vi "Read All FlexiFlow Device States--SubVI.vi"(8 "error in (no error)":errorcluster, 11 "Data Cluster in":T1 {"Flexi-Flow Devices"."Control State"."Control Mode" items=["Bus/RS232"=0, "FLOW-BUS slave"=2, "Valve close"=3, "Controller idle"=4, "Setpoint 100%"=7, "Valve fully open"=8, "Calibration mode"=9, "Setpoint 0%"=12, "RS232"=18, "Valve steering"=20, "Valve safe state"=22]}) -> (0 "error out":errorcluster, 3 "Data Cluster out":T1 {"Flexi-Flow Devices"."Control State"."Control Mode" items=["Bus/RS232"=0, "FLOW-BUS slave"=2, "Valve close"=3, "Controller idle"=4, "Setpoint 100%"=7, "Valve fully open"=8, "Calibration mode"=9, "Setpoint 0%"=12, "RS232"=18, "Valve steering"=20, "Valve safe state"=22]})   [LabVIEW 2025]
uses:
  phlair-shared-libraries/Modbus Flexi-Flow API/Bronkhorst Flexi-Flow ModbusTCP API.lvlib
  phlair-shared-libraries/Modbus Flexi-Flow API/Control Function Values--enum.ctl
  FlexiFlowInterface/Modbus Flexi-Flow Controls--cluster.ctl
  <vilib>/Plasmionique/MB Master/MB_Master_TCP/MB_Master_TCP.lvclass
  FlexiFlowInterface/Modbus Flexi-Flow Measure State--cluster.ctl
  FlexiFlowInterface/Modbus Flexi-Flow State--cluster.ctl
  FlexiFlowInterface/Module Data--cluster.ctl
  phlair-shared-libraries/Modbus Flexi-Flow API/Control Mode--enum.ctl
  FlexiFlowInterface/Device Type--enum.ctl
  FlexiFlowInterface/Modbus TCP Connection Settings--cluster.ctl
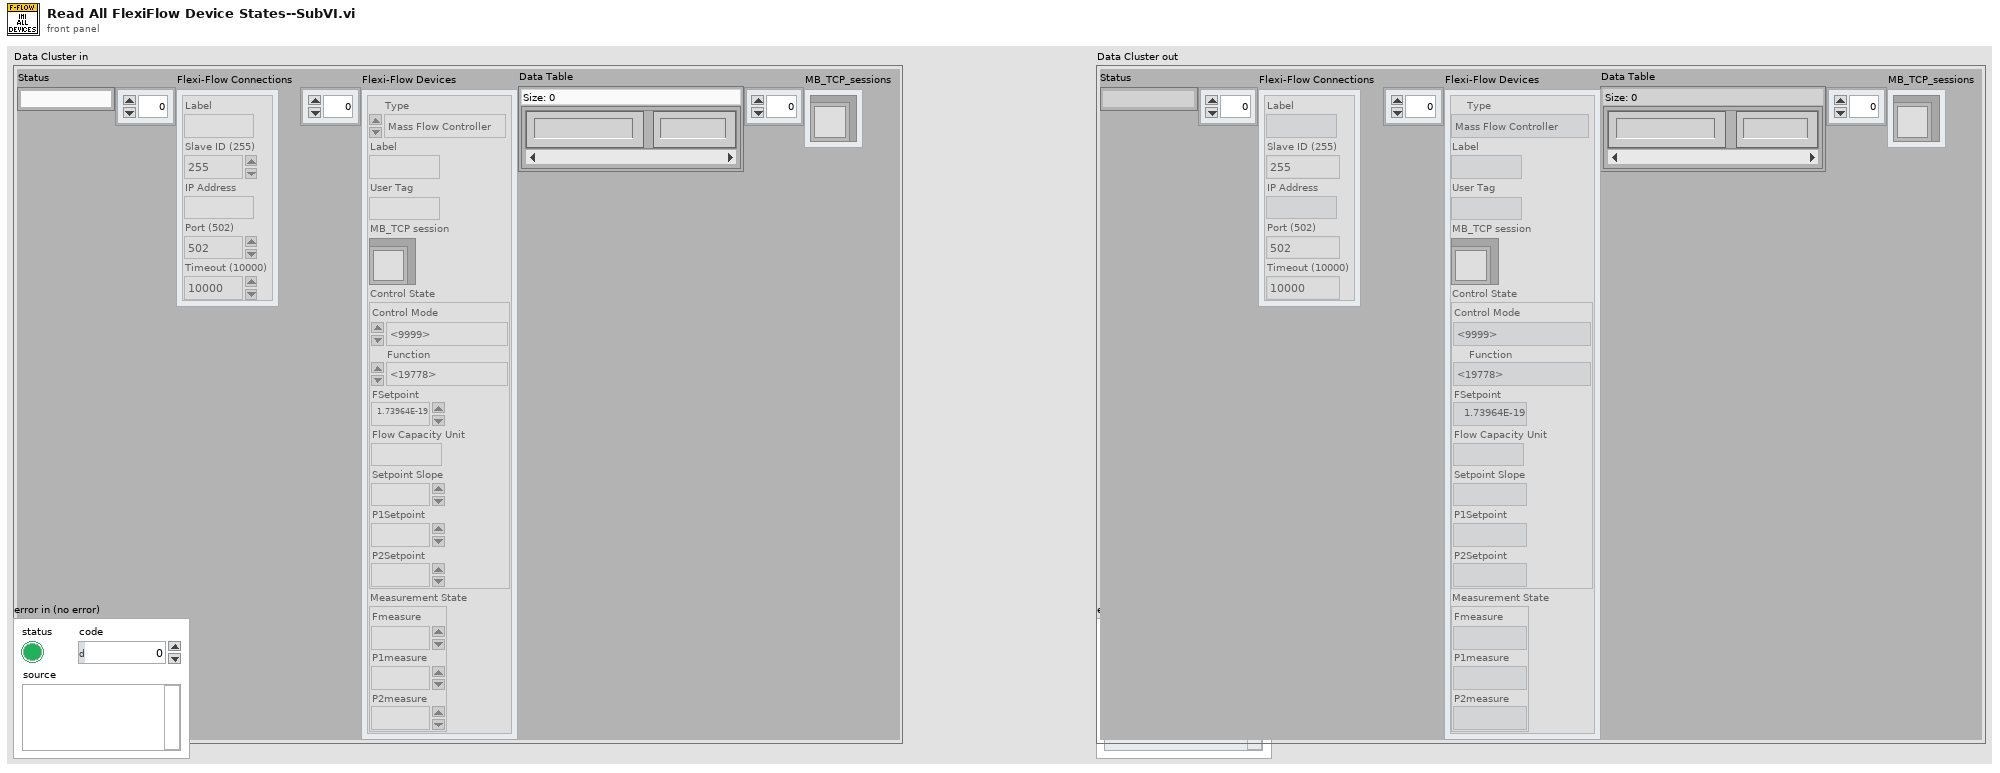
[diagram p1: front panel]
types:
  T1 = typedef "FlexiFlowInterface.lvlib/Module Data--cluster.ctl" = cluster{"Status":string, "Flexi-Flow Connections":T2[], "Flexi-Flow Devices":T3[], "Data Table":map{string, dbl}, "MB_TCP_sessions":refnum<class "MB_Master_TCP.lvclass">[]}
  T2 = typedef "FlexiFlowInterface.lvlib/Modbus TCP Connection Settings--cluster.ctl" = cluster{"Label":string, "Slave ID (255)":u8, "IP Address":string, "Port (502)":u16, "Timeout (10000)":i32}
  T3 = typedef "FlexiFlowInterface.lvlib/Modbus Flexi-Flow State--cluster.ctl" = cluster{"Type":T4, "Label":string, "User Tag":string, "MB_TCP session":refnum<class "MB_Master_TCP.lvclass">, "Control State":T5, "Measurement State":T8}
  T4 = typedef "FlexiFlowInterface.lvlib/Device Type--enum.ctl" = enum16{"Mass Flow Controller", "Mass Flow Meter"}
  T5 = typedef "FlexiFlowInterface.lvlib/Modbus Flexi-Flow Controls--cluster.ctl" = cluster{"Control Mode":T6, "Function":T7, "FSetpoint":sgl, "Flow Capacity Unit":string, "Setpoint Slope":u16, "P1Setpoint":sgl, "P2Setpoint":sgl}
  T6 = typedef "Bronkhorst Flexi-Flow ModbusTCP API.lvlib/Control Mode--enum.ctl" = u16
  T7 = typedef "Bronkhorst Flexi-Flow ModbusTCP API.lvlib/Control Function Values--enum.ctl" = enum16{"Flow", "Upstream pressure", "Downstream pressure", "Flow with upstream pressure limit", "Flow with downstream pressure limit", "Upstream pressure with flow limit", "Downstream pressure with flow limit"}
  T8 = typedef "FlexiFlowInterface.lvlib/Modbus Flexi-Flow Measure State--cluster.ctl" = cluster{"Fmeasure":dbl, "P1measure":sgl, "P2measure":sgl}
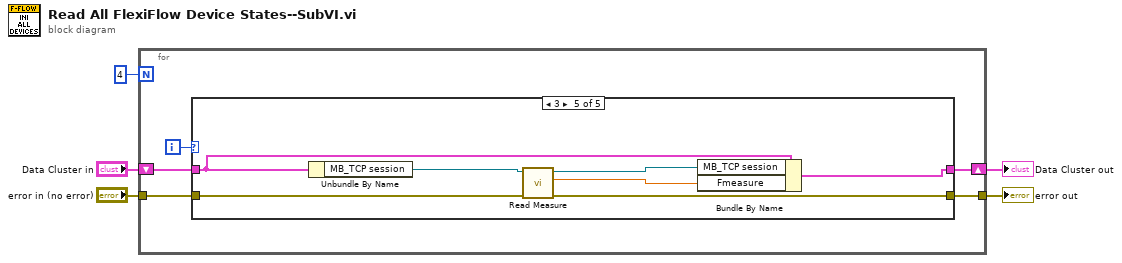
[diagram p0: block diagram]
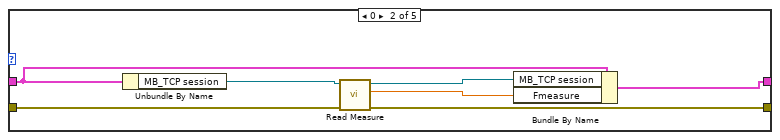
[diagram p3: hidden frame]
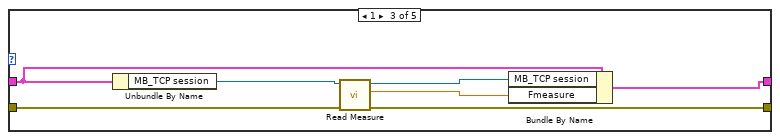
[diagram p4: hidden frame]
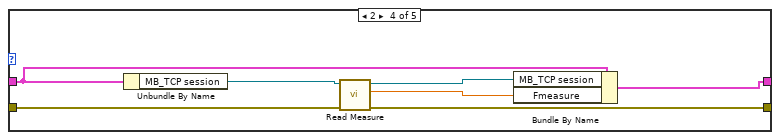
[diagram p5: hidden frame]
diagram:
  n1 = for {
    N: 4 -> [_]
    shift-right: [w9] -> w4
    shift-left: "Data Cluster in" -> [w8]
    tunnel: "error in (no error)" -> [w7]
    tunnel: [w10] -> w5
    i -> [w6]
    n2 = case shown="3" w6 {
      tunnel: [w12 w13 w20 w27 w34] -> w10
      tunnel: [w11 w19 w26 w33 w40] -> w9
      tunnel: w8 -> [w11 w18 w25 w32 w39]
      tunnel: w7 -> [w12 w14 w21 w28 w35]
      frame Default {
      }
      frame 0 {
        n3 = Unbundle By Name(w18) -> ("MB_TCP session"=w17:refnum<class "MB_Master_TCP.lvclass">)
        n4 = call "Read Measure.vi"("error in"=w14, "MB_TCP session in"=w17) -> ("error out"=w13:errorcluster, "Value"=w15:sgl, "MB session out"=w16:refnum<class "MB_Master_TCP.lvclass">)  [unwired: 7 in]
        n5 = Bundle By Name(cluster=w18, "MB_TCP session"=w16, "Fmeasure"=w15) -> (w19:T1)
      }
      frame 1 {
        n6 = Unbundle By Name(w25) -> ("MB_TCP session"=w24:refnum<class "MB_Master_TCP.lvclass">)
        n7 = call "Read Measure.vi"("error in"=w21, "MB_TCP session in"=w24) -> ("error out"=w20:errorcluster, "Value"=w22:sgl, "MB session out"=w23:refnum<class "MB_Master_TCP.lvclass">)  [unwired: 7 in]
        n8 = Bundle By Name(cluster=w25, "MB_TCP session"=w23, "Fmeasure"=w22) -> (w26:T1)
      }
      frame 2 {
        n9 = Unbundle By Name(w32) -> ("MB_TCP session"=w31:refnum<class "MB_Master_TCP.lvclass">)
        n10 = call "Read Measure.vi"("error in"=w28, "MB_TCP session in"=w31) -> ("error out"=w27:errorcluster, "Value"=w29:sgl, "MB session out"=w30:refnum<class "MB_Master_TCP.lvclass">)  [unwired: 7 in]
        n11 = Bundle By Name(cluster=w32, "MB_TCP session"=w30, "Fmeasure"=w29) -> (w33:T1)
      }
      frame 3 {
        n12 = Unbundle By Name(w39) -> ("MB_TCP session"=w38:refnum<class "MB_Master_TCP.lvclass">)
        n13 = call "Read Measure.vi"("error in"=w35, "MB_TCP session in"=w38) -> ("error out"=w34:errorcluster, "Value"=w36:sgl, "MB session out"=w37:refnum<class "MB_Master_TCP.lvclass">)  [unwired: 7 in]
        n14 = Bundle By Name(cluster=w39, "MB_TCP session"=w37, "Fmeasure"=w36) -> (w40:T1)
      }
    }
  }
  "error out" <- w5
  "Data Cluster out" <- w4
